vi "Movement pattern count (SubVI).vi"(0 "Transition Array":i32[](array[numeric]), 2 "Movement patterns":string[](array[string])) -> (7 "Movement Count":i32)   [LabVIEW 2013]
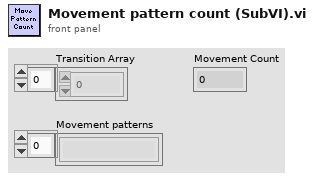
[diagram p1: front panel]
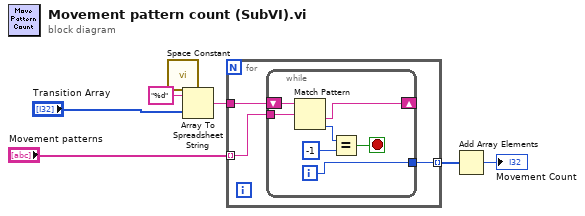
[diagram p0: block diagram]
diagram:
  n1 = call <vilib>:"Space Constant.vi"() -> ("String"=w3:string)
  n2 = Array To Spreadsheet String(delimiter (Tab)=w3, array="Transition Array", 3:"%d" ("format string")) -> (spreadsheet string=w4:string)
  n3 = for {
    tunnel: w4 -> [w10]
    tunnel: "Movement patterns" -> [w9] mode=indexing
    tunnel: [w8] -> w6 mode=indexing
    n4 = while {
      tunnel: w9 -> [w17]
      shift-right: [w15] -> _
      shift-left: w10 -> [w16]
      tunnel: [w11] -> w8
      i -> [w11]
      stop <- w12 stop-if-true
      n5 = Match Pattern(string=w16, regular expression=w17) -> (after substring=w15:string, offset past match=w14:i32)  [unwired: 1 in, 2 out]
      n6 = Equal?(x=w14, y=-1) -> (x = y?=w12:bool)
    }
  }
  n7 = Add Array Elements(numeric array=w6) -> (sum=→"Movement Count":i32)
